vi "Clean Temp Files.vi"(8 "error in (no error)":errorcluster, 10 "Retain Project?":bool, 11 "Builder in":refnum<class "Builder.lvclass">) -> (0 "error out":errorcluster, 3 "Builder out":refnum<class "Builder.lvclass">)   [LabVIEW 2019, in "Builder.lvclass"]
uses:
  Builder.lvclass
  Builder.lvclass/Builder.ctl
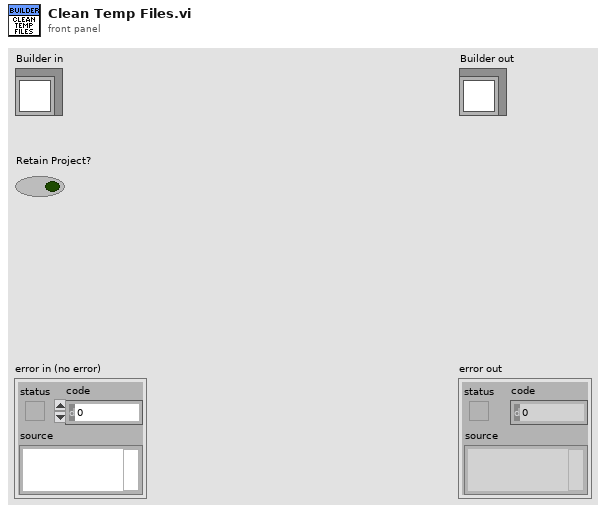
[diagram p1: front panel]
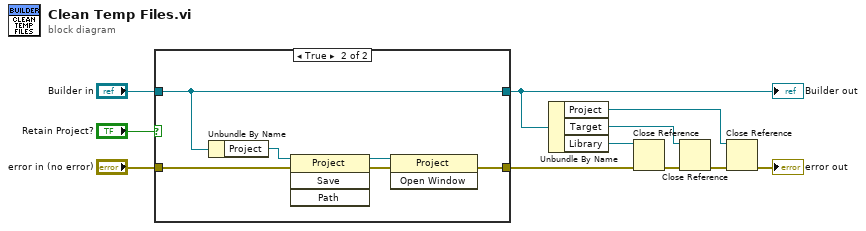
[diagram p0: block diagram]
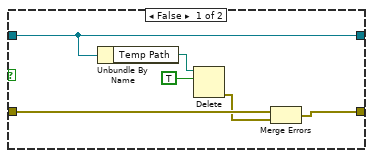
[diagram p2: hidden frame]
diagram:
  n1 = case shown="True" "Retain Project?" {
    tunnel: [w13 w18] -> w11
    tunnel: [w16 w21] -> w7
    tunnel: "Builder in" -> [w16 w21]
    tunnel: "error in (no error)" -> [w14 w19]
    frame False {
      n2 = Unbundle By Name(w16) -> ("Temp Path"=w15:path)
      n3 = Delete(path (use dialog)=w15, entire hierarchy (F)=TRUE) -> (error out=w12:errorcluster)  [unwired: 3 in, 2 out]
      n4 = Merge Errors(w14, w12) -> (w13:errorcluster)
    }
    frame True {
      n5 = Unbundle By Name(w21) -> ("Project"=w20:refnum<vi>)
      n6 = invoke class="Project" method="Save"(reference=w20, error in=w19) -> (reference out=w22:refnum<vi>, error out=w23:errorcluster)  [unwired: 2 in, 2 out]
      n7 = invoke class="Project" method="Open Window"(reference=w22, error in=w23) -> (error out=w18:errorcluster)  [unwired: 1 in, 2 out]
    }
  }
  "Builder out" <- w7
  n8 = Unbundle By Name(w7) -> ("Project"=w1:refnum<vi>, "Target"=w3:refnum<vi>, "Library"=w5:refnum<vi>)
  n9 = Close Reference(reference=w5, error in (no error)=w11) -> (error out=w6:errorcluster)
  n10 = Close Reference(reference=w3, error in (no error)=w6) -> (error out=w4:errorcluster)
  n11 = Close Reference(reference=w1, error in (no error)=w4) -> (error out=→"error out":errorcluster)
